vi "OPC Set Properties Name.vi"(8 "error in (no error)":errorcluster, 9 "name":string, 10 "item node ID":T1, 11 "Refnum in":T4) -> (0 "error out":errorcluster, 3 "OPC Property cluster":T3)   [LabVIEW 2018]
uses:
  <vilib>/OPCUA/controls/NodeId.ctl
  <vilib>/OPCUA/controls/OPC UA Server Refnum.ctl
  <vilib>/OPCUA/controls/OPC UA Variable Node Refnum.ctl
  <vilib>/OPCUA/controls/Data Type.ctl
  <vilib>/OPCUA/NI OPC UA Server.lvlib
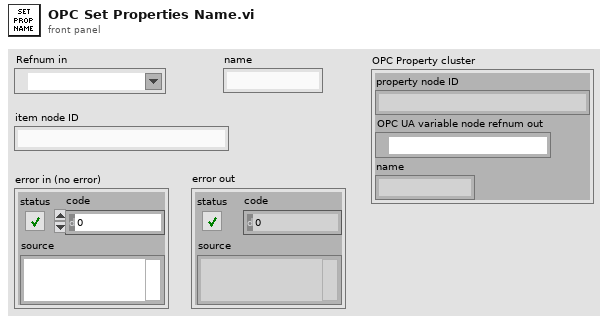
[diagram p1: front panel]
types:
  T1 = typedef "NodeId.ctl" = string
  T2 = typedef "OPC UA Variable Node Refnum.ctl" = refnum<k21>
  T3 = cluster{"property node ID":T1, "OPC UA variable node refnum out":T2, "name":string}
  T4 = typedef "OPC UA Server Refnum.ctl" = refnum<k21>
  T5 = typedef "Data Type.ctl" = u16
  T6 = cluster{"name":string, "data type":T5, "access level":u16, "description":string}
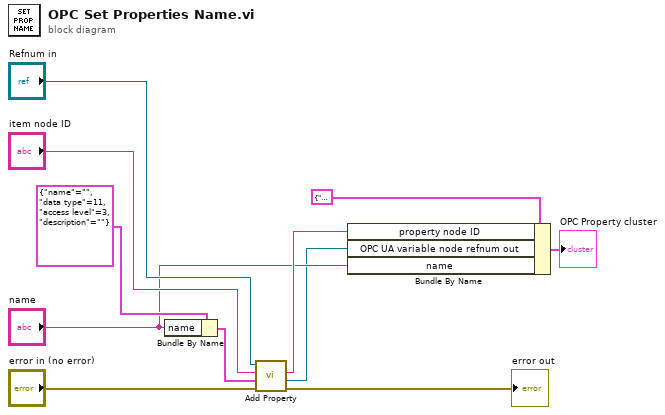
[diagram p0: block diagram]
diagram:
  n1 = Bundle By Name(cluster=T6 {"name"="", "data type"=11, "access level"=3, "description"=""} ("property"), "name"="name") -> (w8:T6)
  n2 = call <vilib>:"Add Property.vi"("error in (no error)"="error in (no error)", "property"=w8, "item node ID"="item node ID", "OPC UA server refnum in"="Refnum in") -> ("error out"=→"error out":errorcluster, "OPC UA variable node refnum out"=w2:T2, "property node ID"=w4:T1)  [unwired: 3 in, 1 out]
  n3 = Bundle By Name(cluster=T3 {"property node ID"="", "OPC UA variable node refnum out"="", "name"=""}, "property node ID"=w4, "OPC UA variable node refnum out"=w2, "name"="name") -> (→"OPC Property cluster":T3)
